vi "lv_icon.vi"(8 "error in (no error)":errorcluster, 9 "BW icon in":T1, 10 "Color icon in":T1, 11 "_IconEditorInterface in":refnum<class "IconEditorInterface.lvclass">) -> (0 "error out":errorcluster, 1 "Color icon out":T1, 2 "BW icon out":T1, 3 "_IconEditorInterface out":refnum<class "IconEditorInterface.lvclass">, 4 "Error code out":i32)   [LabVIEW 2021, in "IconEditorInterface.lvlib" / "IconEditorInterface.lvclass"]
uses:
  IconEditorInterface.lvclass
  <vilib>/picture/picture.llb/imagedata.ctl
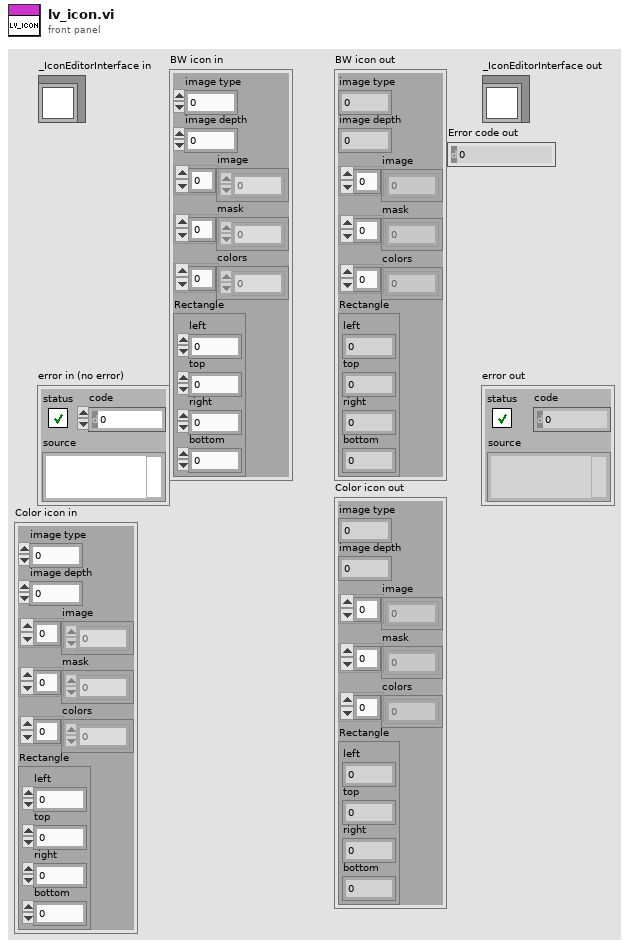
[diagram p1: front panel]
types:
  T1 = typedef "imagedata.ctl" = cluster{"image type":i32, "image depth":i32, "image":u8[], "mask":u8[], "colors":u32[], "Rectangle":cluster{"left":i16, "top":i16, "right":i16, "bottom":i16}}
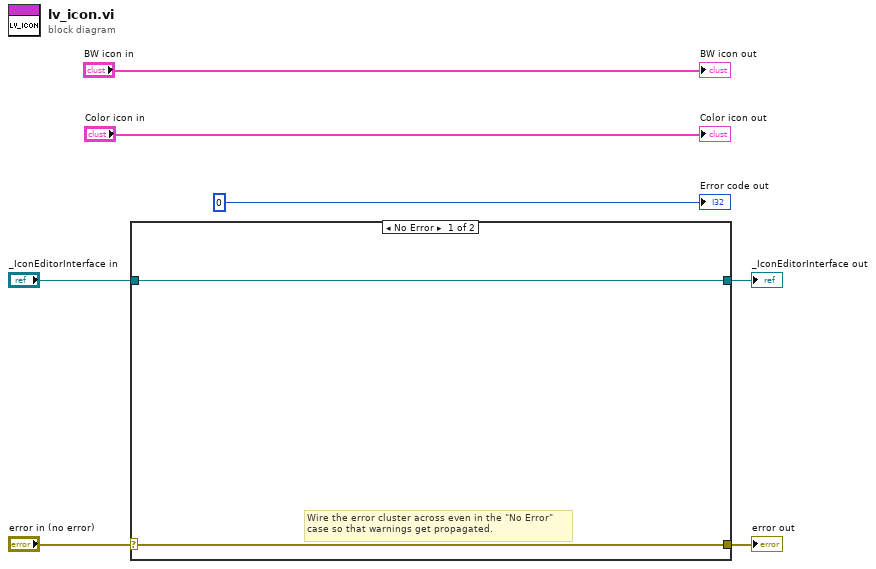
[diagram p0: block diagram]
diagram:
  n1 = case shown="No Error" "error in (no error)" {
    selector: "error in (no error)" -> [w8 w11]
    tunnel: [w8 w11] -> w6
    tunnel: [w9 w10] -> w4
    tunnel: "_IconEditorInterface in" -> [w9 w10]
    frame No Error {
      # "Wire the error cluster across even in the \"No Error\"\ncase so that warnings get propagated."
    }
    frame Error {
    }
  }
  "error out" <- w6
  "_IconEditorInterface out" <- w4
  "BW icon out" <- "BW icon in"
  "Color icon out" <- "Color icon in"
  "Error code out" <- 0 ("code")
